vi "Get Step Count.vi"(8 "error in (no error)":errorcluster, 11 "Macro in":refnum<class "Macro.lvclass">) -> (0 "error out":errorcluster, 2 "Step Count":i32, 3 "Macro out":refnum<class "Macro.lvclass">)   [LabVIEW 2020, in "MacroAssert.lvlib" / "Macro.lvclass"]
uses:
  Macro.lvclass
  Step/Step.lvclass
  Macro.lvclass/Macro.ctl
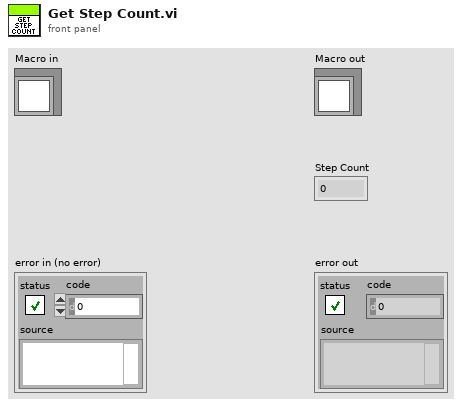
[diagram p1: front panel]
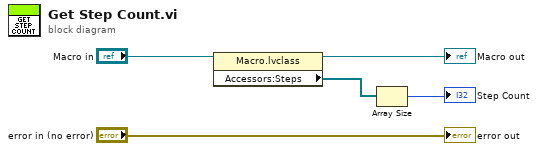
[diagram p0: block diagram]
diagram:
  n1 = property class="Macro.lvclass"(reference="Macro in") -> (reference out=→"Macro out":refnum<class "Macro.lvclass">, "Accessors:Steps"=w1:refnum<class "Step.lvclass">[])  [unwired: 1 in, 1 out]
  n2 = Array Size(array=w1) -> (size(s)=→"Step Count":i32)
  "error out" <- "error in (no error)"
